vi "note.vi"() -> (2 "out":string)   [LabVIEW 2012]
panel:
  out "Canceled?":bool
  in  "Ctl Refnum":refnum<vi>
  in  "Cancel Button":bool
  in  "OK Button":bool
  in  "note":string caption="Примечание"
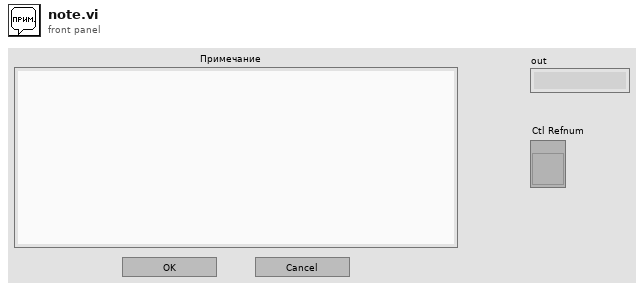
[diagram p1: front panel]
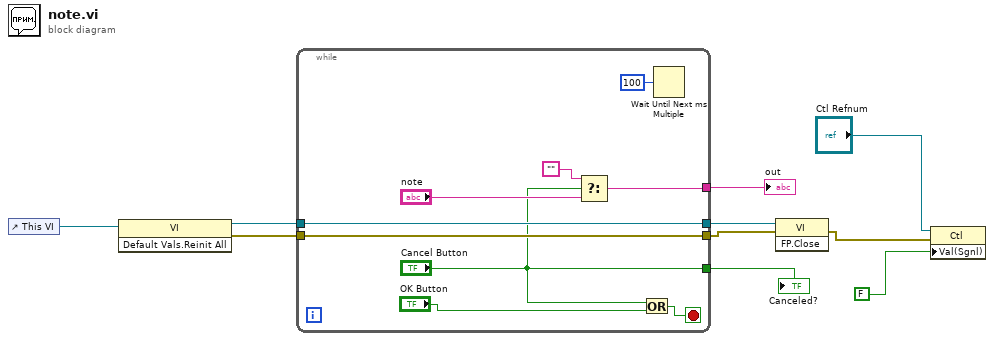
[diagram p0: block diagram]
diagram:
  n1 = control-ref of="This VI"() -> (w9:refnum<vi>)
  n2 = invoke class="VI" method="Default Vals.Reinit All"(reference=w9) -> (reference out=w7:refnum<vi>, error out=w8:errorcluster)  [unwired: 2 in, 1 out]
  n3 = while {
    tunnel: [w15] -> w10
    tunnel: w8 -> [w12]
    tunnel: w7 -> [w13]
    tunnel: [w13] -> w6
    tunnel: [w12] -> w5
    tunnel: ["Cancel Button"] -> w1
    stop <- w18 stop-if-true
    n4 = Select(t="", s="Cancel Button", f="note") -> (s? t:f=w15:string)
    n5 = Or(x="Cancel Button", y="OK Button") -> (x .or. y?=w18:bool)
    n6 = Wait Until Next ms Multiple(millisecond multiple=u32 100) -> ()  [unwired: 1 out]
  }
  "out" <- w10
  "Canceled?" <- w1
  n7 = invoke class="VI" method="FP.Close"(reference=w6, error in=w5) -> (error out=w2:errorcluster)  [unwired: 1 in, 2 out]
  n8 = property class="Ctl"(reference="Ctl Refnum", error in=w2, "Val(Sgnl)"=FALSE) -> ()  [unwired: 2 out]
